vi "_Dialog_parameters (SubVI).vi"() -> (3 "Cancelled?":bool)   [LabVIEW 2017]
doc: "Use this template to create a dialog box with event handling."
panel:
  in  "Tab2":T1(tab)
  in  "Encoder2CurrData":i64 caption="Текущее значение счетчика энкодера 2"
  in  "Encoder2ScalingFactor":i32=100 caption="Масштабный коэффициент, нм/имп"
  in  "Encoder2AInv":bool
  in  "Encoder2BInv":bool
  in  "Encoder2ZInv":bool
  in  "Encoder2ZEn":bool
  in  "Encoder2En":bool
  in  "Encoder1CurrData":i64 caption="Текущее значение счетчика энкодера 1"
  in  "Encoder1ScalingFactor":i32=100 caption="Масштабный коэффициент, нм/имп"
  in  "Encoder1AInv":bool
  in  "Encoder1BInv":bool
  in  "Encoder1ZInv":bool
  in  "Encoder1ZEn":bool
  in  "Encoder1En":bool
  in  "PulseCurrData":i64 caption="Текущее значение счетчика импульсов"
  in  "PulseSensitivity":u16(ring)=1 caption="Тип запуска для режима" items=["Фронт"=1, "Срез"=2, "Оба"=3]
  in  "PulseScalingFactor":i32=100 caption="Масштабный коэффициент, нм/имп"
  in  "PulseInput":T2(ring) caption="Вход импульса запуска"
  in  "PulseCounterEn":bool
  in  "EncoderSync":i64=1 caption="Величина \"К\""
  out "NumOfRuns":i32=994875 caption="Счетчик количества запусков цикла"
  in  "DataEncodersParam2":enum16{"Encoder1CurrData", "PulseCurrData"}(ring) caption="Параметры поля \"Encoders Param 2\""
  in  "EncoderNum":u16(ring)=1 caption="Номер энкодера для режима \"Энкодер\"" items=["1"=1, "2"=2]
  in  "SyncMode":u16(ring)=1 caption="Источник синхронизации" items=["Внутренний таймер"=1, "Энкодер"=2, "Внешний импульс"=3]
  in  "DataEncodersParam1":enum16{"Encoder1CurrData", "PulseCurrData"}(ring) caption="Параметры поля \"Encoders Param 1\""
  in  "TimerSyncInt":i32=10000 caption="Интервал времени запуска цикла"
  in  "FPGA1ExtRAMBuffEn":bool=TRUE
  in  "FPGA0ExtRAMBuffEn":bool=TRUE
  in  "Meas":bool=TRUE
  in  "Cancel":bool
  in  "OK":bool
  # "Энкодер 1"
  # "Энкодер 2"
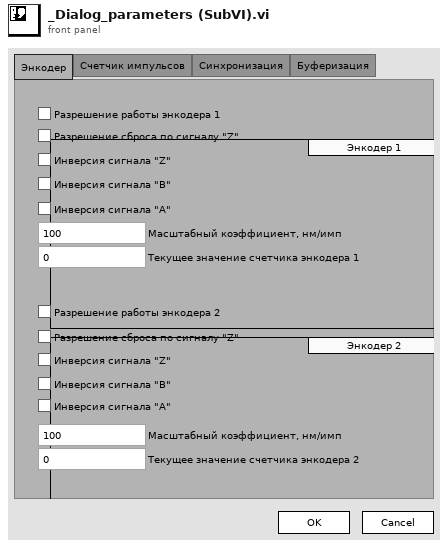
[diagram p1: front panel]
types:
  T1 = enum32{"Энкодер", "Счетчик импульсов", "Синхронизация", "Буферизация"}
  T2 = enum16{"X17 вход 1", "X17 вход 2", "X17 вход 3", "X18 вход 1", "X18 вход 2", "X18 вход 3"}
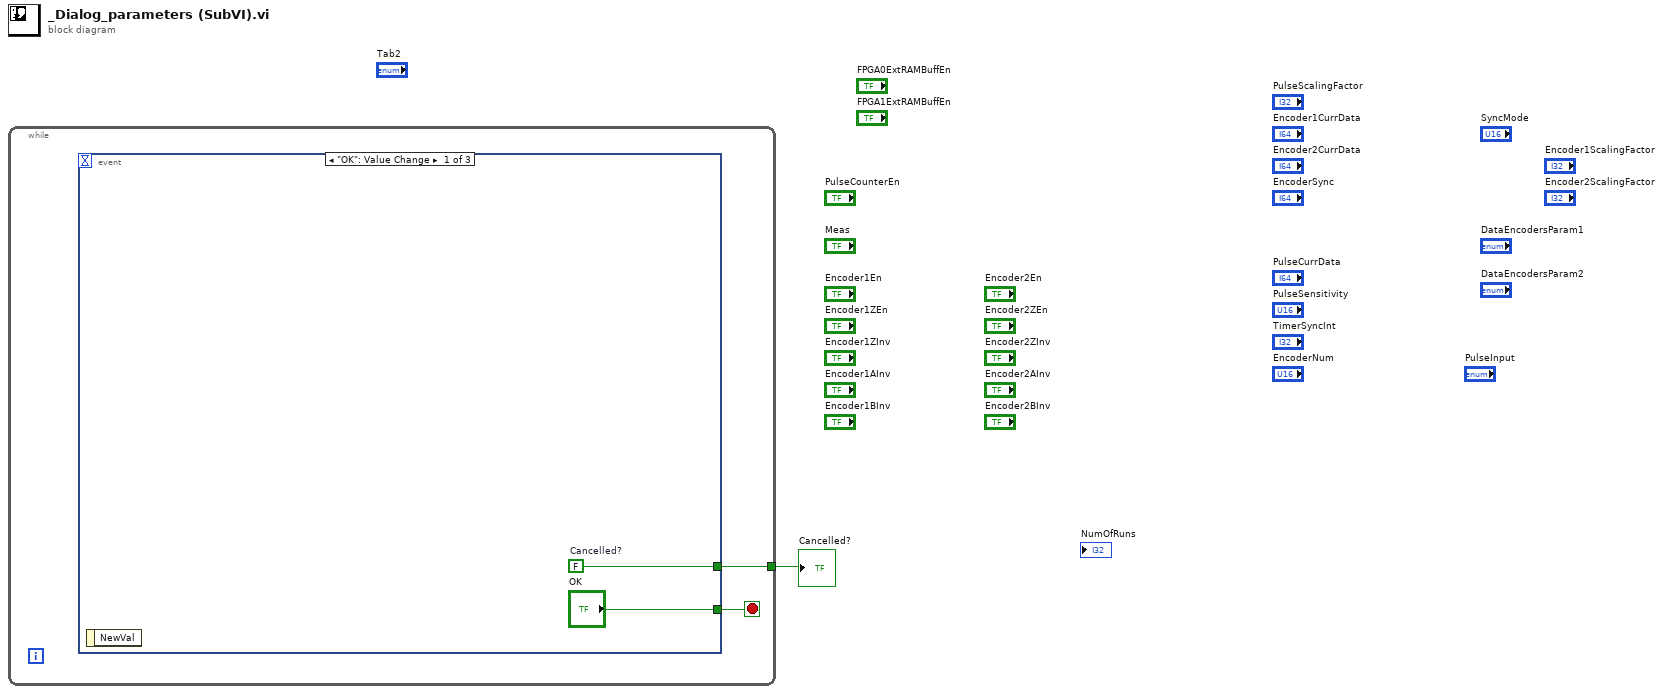
[diagram p0: block diagram]
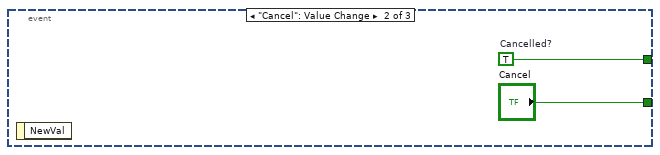
[diagram p2: hidden frame]
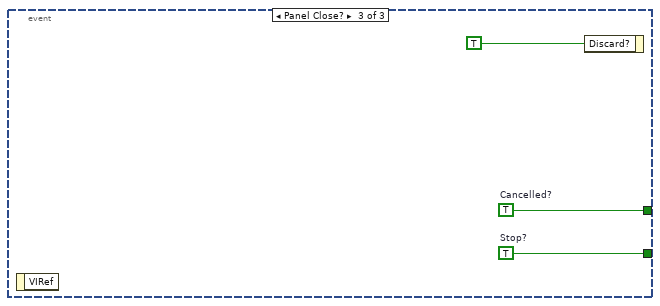
[diagram p3: hidden frame]
diagram:
  n1 = while {
    tunnel: [w2] -> w1
    stop <- w3 stop-if-true
    n2 = event shown="[0] \"OK\": Value Change" {
      selector: _ -> [_ _ _]
      dyn-events: _ -> [_ _ _]
      timeout: _ -> [_ _ _]
      tunnel: ["OK" "Cancel" w9] -> w3
      tunnel: [w5 w7 w8] -> w2
      event "OK": Value Change {
        w5 = FALSE  # Cancelled?
        n3 = event-data() -> ()  [unwired: 1 in, 1 out]
      }
      event "Cancel": Value Change {
        w7 = TRUE  # Cancelled?
        n4 = event-data() -> ()  [unwired: 1 in, 1 out]
      }
      event Panel Close? {
        w8 = TRUE  # Cancelled?
        w9 = TRUE  # Stop?
        n5 = event-data() -> ()  [unwired: 1 in, 1 out]
        n6 = event-data("Discard?"=TRUE) -> ()  [unwired: 1 in, 1 out]
      }
    }
  }
  "Cancelled?" <- w1
